vi "Enqueue.vi"(7 "Priority (f)":bool, 8 "ErrorArray In":errorcluster[](array[cluster]), 9 "Data":variant, 10 "Msg":string) -> (0 "ErrorArray Out":errorcluster[](array[cluster]))   [LabVIEW 2014, in "Bus.lvlib" / "NISTBus.lvclass"]
uses:
  NISTBus.lvclass
  Framework/MsgQueue/TypeDef/MsgQueue.ctl
  <userlib>/NIST/NISTErrorLib/NISTErrorLib.lvlib
  Framework/TestFramework.lvlib
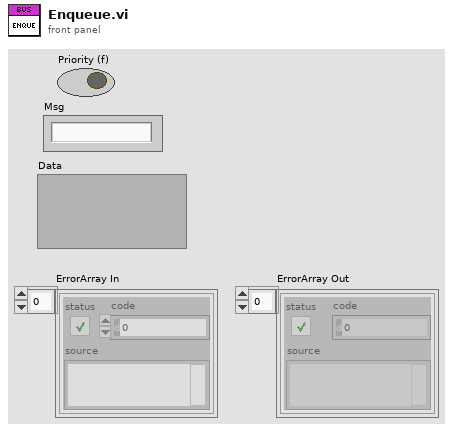
[diagram p1: front panel]
types:
  T1 = typedef "TestFramework.lvlib/MsgQueue.ctl" = cluster{"Msg":string, "Data":variant}
  T2 = typedef "TestFramework.lvlib/QueRef.ctl" = refnum<queue>
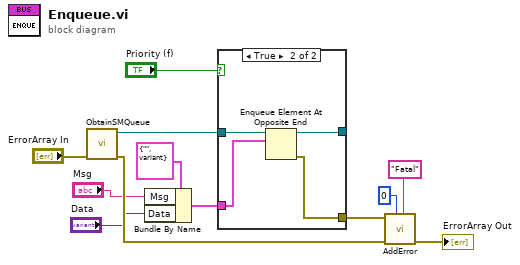
[diagram p0: block diagram]
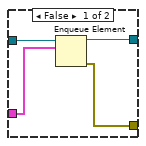
[diagram p2: hidden frame]
diagram:
  n1 = call "ObtainSMQueue.vi"("ErrorArray In"="ErrorArray In") -> ("ErrorArray Out"=w8:errorcluster[], "QueRef"=w10:T2)  [unwired: 9 in]
  n2 = Bundle By Name(cluster=T1 {"Msg"="", "Data"=variant} ("MsgQueue"), "Msg"="Msg", "Data"="Data") -> (w4:T1)
  n3 = case shown="True" "Priority (f)" {
    tunnel: w10 -> [w16 w20]
    tunnel: [w15 w19] -> _
    tunnel: w4 -> [w14 w18]
    tunnel: [w13 w17] -> w3
    frame False {
      n4 = Enqueue Element(queue=w16, element=w14) -> (queue out=w15:T2, error out=w13:errorcluster)  [unwired: 2 in, 1 out]
    }
    frame True {
      n5 = Enqueue Element At Opposite End(queue=w20, element=w18) -> (queue out=w19:T2, error out=w17:errorcluster)  [unwired: 2 in, 1 out]
    }
  }
  n6 = call <userlib>:"AddError.vi"("Severity"="Fatal", "Priority"=u8 0, "ErrorArray"=w8, "error in (no error)"=w3) -> ("ErrorArray"=→"ErrorArray Out":errorcluster[])  [unwired: 6 in, 1 out]
